vi "Step Move.vi"(8 "Error In":errorcluster, 9 "Delta Y":dbl, 10 "Delta X":dbl, 11 "Address/Port in":i16) -> (0 "Error Out":errorcluster, 3 "Address/Port out":i16)   [LabVIEW 2014]
doc: "Move the motors \"X\" and \"Y\" respectively of Delta X and Delta Y steps"
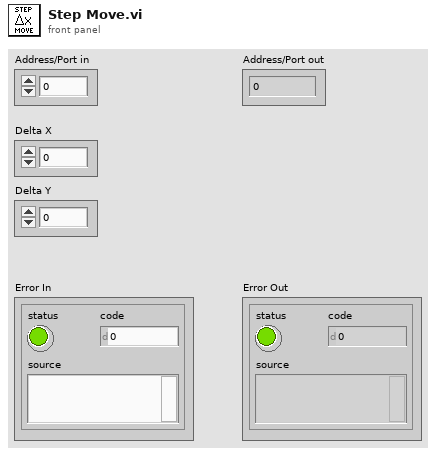
[diagram p1: front panel]
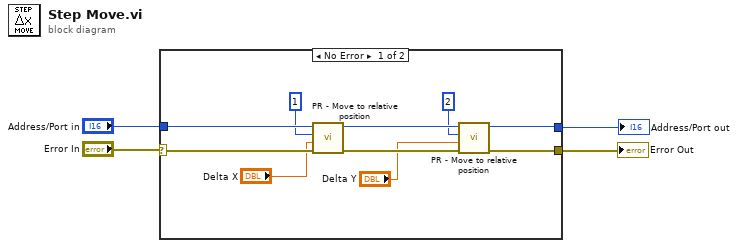
[diagram p0: block diagram]
diagram:
  n1 = case shown="No Error" "Error In" {
    selector: "Error In" -> [w14 w16]
    tunnel: [w11 w16] -> w3
    tunnel: "Address/Port in" -> [w13 w15]
    tunnel: [w8 w15] -> w1
    frame No Error {
      n2 = call "PR - Move to relative position.vi"("error in"=w14, "Nstep"="Delta X", "Axis  #"=i8 1, "Address / Port"=w13) -> ("error out"=w12:errorcluster, "Address / Port dup"=w10:i16)  [unwired: 3 in, 1 out]
      n3 = call "PR - Move to relative position.vi"("error in"=w12, "Nstep"="Delta Y", "Axis  #"=i8 2, "Address / Port"=w10) -> ("error out"=w11:errorcluster, "Address / Port dup"=w8:i16)  [unwired: 3 in, 1 out]
    }
    frame Error {
    }
  }
  "Error Out" <- w3
  "Address/Port out" <- w1
